vi "MultipleMeasurements.vi"(8 "error in (no error)":errorcluster, 10 "Time in ms (30000)":u32=30000, 11 "VISA resource name":refnum<visa-resource-name>) -> (0 "error out":errorcluster, 1 "Raw output":dbl[](array[numeric]), 2 "output/s":dbl[](array[numeric]), 3 "VISA resource name out":refnum<visa-resource-name>)   [LabVIEW 2017, in "GP22_TDC_Arduinoed.lvlib"]
doc: "Measure the time between triggers and output an array of all these measurements in the given measurement period."
uses:
  GP22_TDC_Arduinoed.lvlib
  Private/ConvertTimes - Array.vi
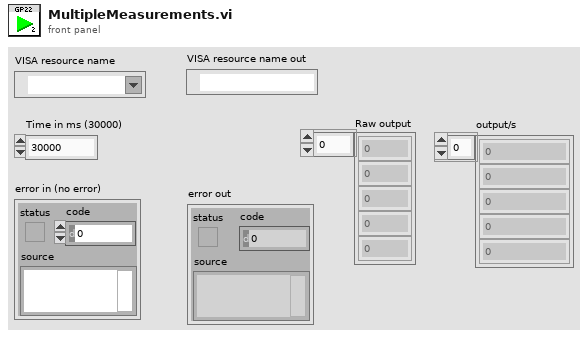
[diagram p1: front panel]
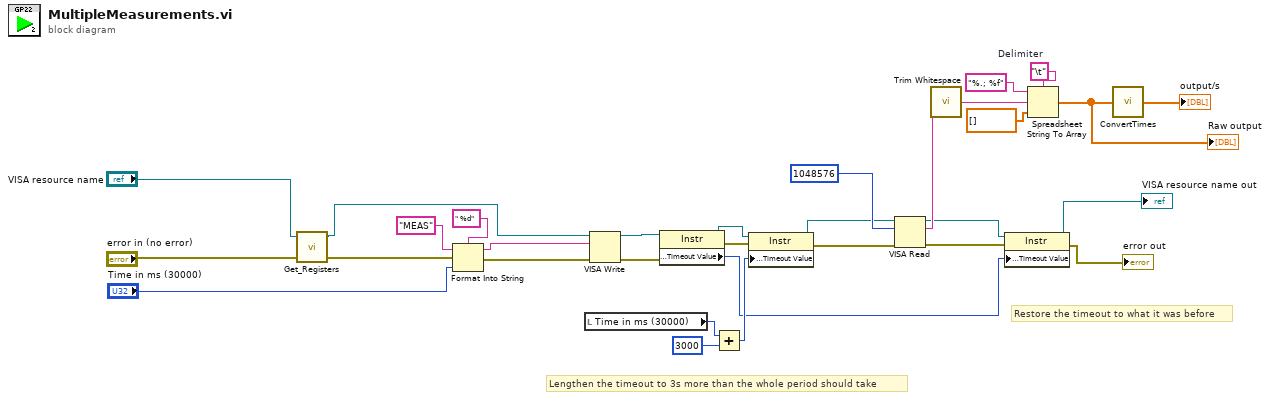
[diagram p0: block diagram]
diagram:
  w26 = "\t"  # Delimiter
  # "Restore the timeout to what it was before"
  # "Lengthen the timeout to 3s more than the whole period should take"
  n1 = call "Get_Registers.vi"("error in (no error)"="error in (no error)", "VISA in"="VISA resource name") -> ("error out"=w3:errorcluster, "VISA out"=w4:refnum<visa-resource-name>)  [unwired: 1 in, 1 out]
  n2 = Format Into String(format string=" %d", initial string="MEAS" ("command"), error in=w3, "Time in ms (30000)") -> (resulting string=w28:string, error out=w31:errorcluster)
  n3 = local read "Time in ms (30000)"() -> (w15:u32)
  n4 = VISA Write(VISA resource name=w4, write buffer=w28, error in (no error)=w31) -> (VISA resource name out=w22:refnum<visa-resource-name>, error out=w21:errorcluster)  [unwired: 1 out]
  n5 = property class="Instr"(reference=w22, error in=w21) -> (reference out=w20:refnum<visa-resource-name>, error out=w19:errorcluster, "General Settings:Timeout Value"=w9:u32)
  n6 = Add(x=w15, y=3000) -> (x+y=w16:u32)
  n7 = property class="Instr"(reference=w20, error in=w19, "General Settings:Timeout Value"=w16) -> (reference out=w18:refnum<visa-resource-name>, error out=w17:errorcluster)
  n8 = VISA Read(VISA resource name=w18, byte count=u32 1048576, error in (no error)=w17) -> (VISA resource name out=w13:refnum<visa-resource-name>, read buffer=w23:string, error out=w12:errorcluster)  [unwired: 1 out]
  n9 = call <vilib>:"Trim Whitespace.vi"("string"=w23) -> ("trimmed string"=w6:string)  [unwired: 1 in]
  n10 = property class="Instr"(reference=w13, error in=w12, "General Settings:Timeout Value"=w9) -> (reference out=→"VISA resource name out":refnum<visa-resource-name>, error out=→"error out":errorcluster)
  n11 = Spreadsheet String To Array(delimiter (Tab)=w26, format string="%.; %f", spreadsheet string=w6, array type (2D Dbl)=dbl[] []) -> (array=w7:dbl[])
  "Raw output" <- w7
  n12 = call-poly "ConvertTimes.vi"("GP22 results"=w7) -> ("Array of times / s"=→"output/s":dbl[])
